vi "6-1.vi"() -> ()   [LabVIEW 2017]
panel:
  out "路径":path
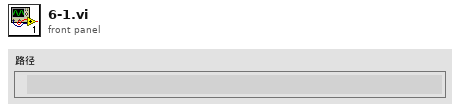
[diagram p1: front panel]
types:
  T1 = enum16{"open", "replace", "create", "open or create", "replace or create", "replace or create with confirmation"}
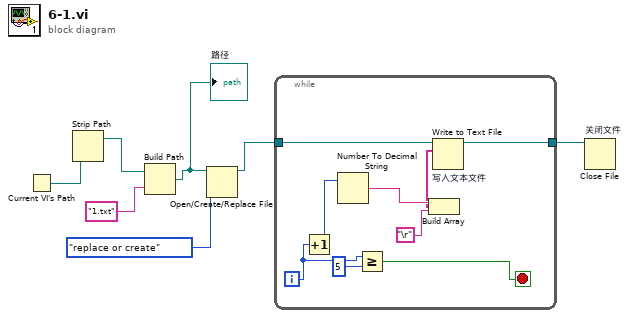
[diagram p0: block diagram]
diagram:
  n1 = Current VI's Path() -> (path=w7:path)
  n2 = Strip Path(path=w7) -> (stripped path=w6:path)  [unwired: 1 out]
  n3 = Build Path(base path=w6, name or relative path="1.txt" ("名称或相对路径")) -> (appended path=w2:path)
  "路径" <- w2
  n4 = Open/Create/Replace File(file path (use dialog)=w2, operation (0:open)=T1."replace or create" ("操作(0:open)")) -> (refnum out=w4:refnum<file>)  [unwired: 4 in, 2 out]
  n5 = while {
    tunnel: w4 -> [w13]
    tunnel: [w8] -> w1
    i -> [w16]
    stop <- w12 stop-if-true
    n6 = Increment(x=w16) -> (x+1=w14:i32)
    n7 = Number To Decimal String(number=w14) -> (decimal integer string=w11:string)  [unwired: 1 in]
    n8 = Greater Or Equal?(x=w16, y=5) -> (x >= y?=w12:bool)
    n9 = Build Array(w11, "\r") -> (w10:string[])
    n10 = Write to Text File "写入文本文件"(file (use dialog)=w13, text=w10) -> (refnum out=w8:refnum<file>)  [unwired: 2 in, 2 out]
  }
  n11 = Close File "关闭文件"(refnum=w1) -> ()  [unwired: 1 in, 2 out]
